vi "Test Strictly Unsupported ISO8601 Strings.vi"(8 "error in (no error)":errorcluster) -> (0 "error out":errorcluster)   [LabVIEW 2017]
uses:
  <vilib>/Utility/file.llb/Read From Spreadsheet File (string).vi
  <vilib>/addons/_JKI Toolkits/Caraya/classes/Assert/Assert False.vi
  <vilib>/addons/_JKI Toolkits/Caraya/classes/Assert/Assert.lvclass
  <vilib>/addons/_JKI Toolkits/Caraya/classes/Test/Test.lvclass
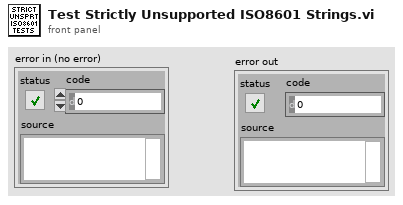
[diagram p1: front panel]
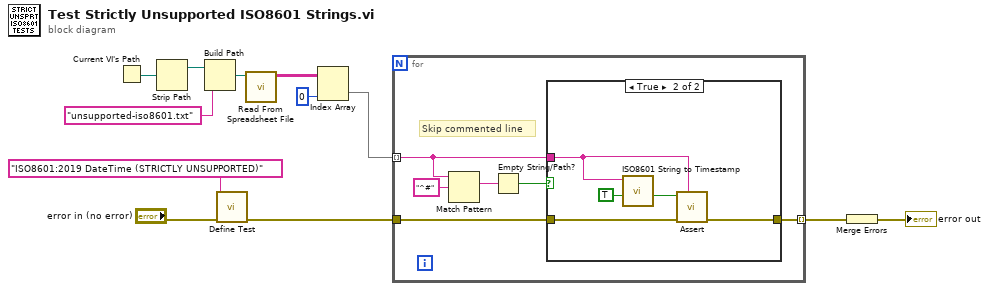
[diagram p0: block diagram]
diagram:
  n1 = Current VI's Path() -> (path=w5:path)
  n2 = Strip Path(path=w5) -> (stripped path=w6:path)  [unwired: 1 out]
  n3 = Build Path(base path=w6, name or relative path="unsupported-iso8601.txt") -> (appended path=w7:path)
  n4 = call <vilib>:"Define Test.vi"("error in (no error)"="error in (no error)", "Label (VI Title)"="ISO8601:2019 DateTime (STRICTLY UNSUPPORTED)") -> ("error out"=w11:errorcluster)  [unwired: 8 in, 1 out]
  n5 = call-poly <vilib>:"Read From Spreadsheet File.vi"("file path (dialog if empty)"=w7) -> ("all rows"=w2:string[][])  [unwired: 6 in, 4 out]
  n6 = Index Array(array=w2, index (col)=0 ("disabled index (col)")) -> (element=w4:string[])  [unwired: 1 in]
  n7 = for {
    tunnel: w4 -> [w16] mode=indexing
    tunnel: [w17] -> w8 mode=indexing
    tunnel: w11 -> [w18]
    # "Skip commented line"
    n8 = Match Pattern(string=w16, regular expression="^#") -> (match substring=w14:string)  [unwired: 1 in, 3 out]
    n9 = Empty String/Path?(string/path=w14) -> (empty?=w13:bool)
    n10 = case shown="True" w13 {
      tunnel: w18 -> [w19 w24]
      tunnel: [w19 w23] -> w17
      tunnel: w16 -> [_ w20]
      frame False {
        # "Skip"
      }
      frame True {
        n11 = call "ISO8601 String to Timestamp.vi"("Strict ISO? (T)"=TRUE, "ISO8601 String"=w20) -> ("valid?"=w21:bool)  [unwired: 7 in, 2 out]
        n12 = call-poly <vilib>:"Assert.vi"("Label"=w20, "error in (no error)"=w24, "False?"=w21) -> ("error out"=w23:errorcluster)  [unwired: 7 in, 1 out]
      }
    }
  }
  n13 = Merge Errors(w8) -> (→"error out":errorcluster)
